vi "Nonredundant Swap Neighborhood.vi"(6 "Number of Machines":i32, 8 "w":i32, 9 "y":i32, 10 "Generate Random indices?":bool, 11 "Schedule in":u16[](array[numeric])) -> (3 "Schedule out":u16[](array[numeric]))   [LabVIEW 2013]
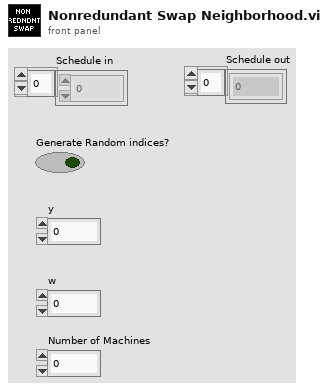
[diagram p1: front panel]
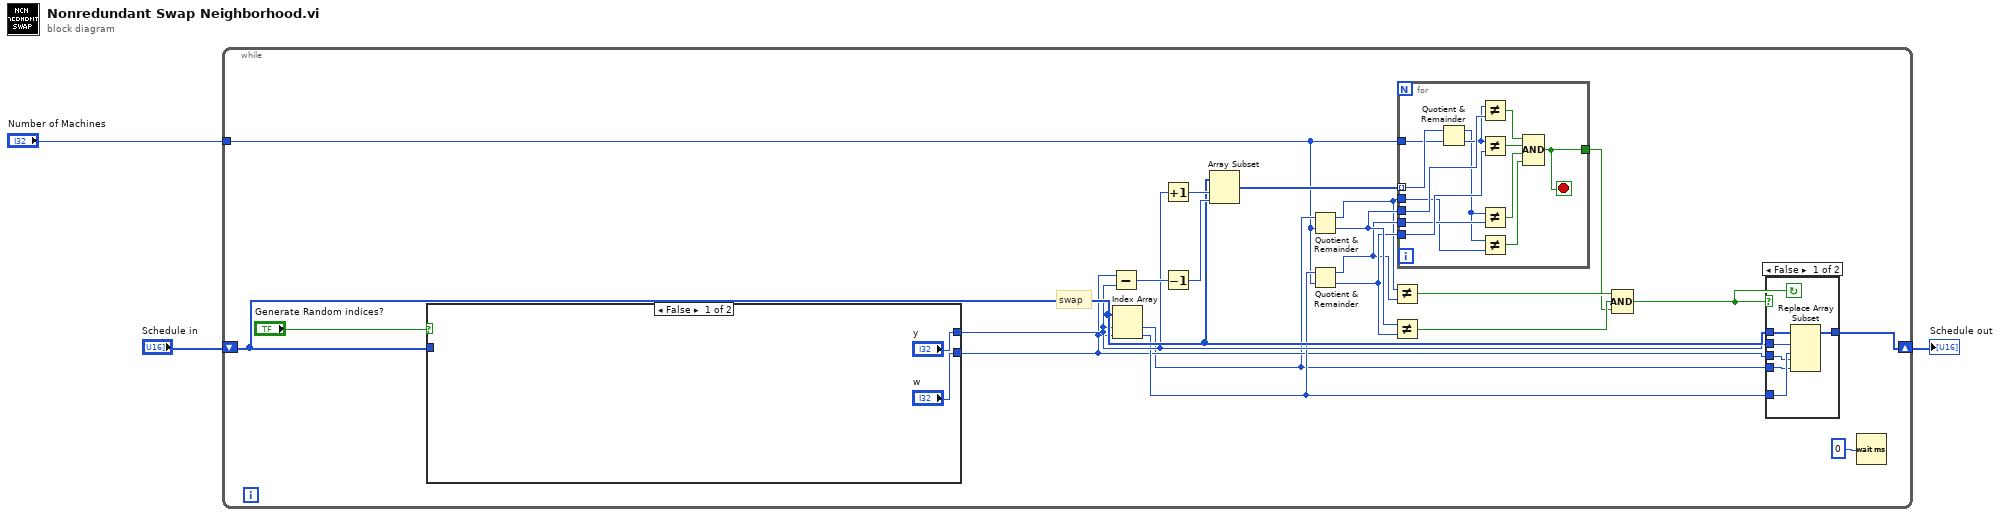
[diagram p0: block diagram]
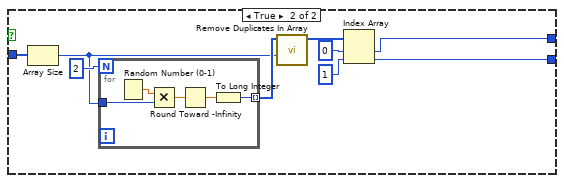
[diagram p2: hidden frame]
diagram:
  n1 = while {
    shift-right: [w11] -> w3
    shift-left: "Schedule in" -> [w12]
    tunnel: "Number of Machines" -> [w6]
    stop <- w13 continue-if-true
    # "swap"
    n2 = case shown="False" "Generate Random indices?" {
      tunnel: w12 -> [_ w32]
      tunnel: ["y" w31] -> w10
      tunnel: ["w" w30] -> w8
      frame False {
      }
      frame True {
        n3 = Array Size(array=w32) -> (size(s)=w28:i32)
        n4 = for {
          N: 2 -> [_]
          tunnel: w28 -> [w37]
          tunnel: [w36] -> w29 mode=indexing
          n5 = Random Number (0-1)() -> (number: 0 to 1=w40:dbl)
          n6 = Multiply(x=w40, y=w37) -> (x*y=w39:dbl)
          n7 = Round Toward -Infinity(1:w39) -> (0:w38:dbl)
          n8 = To Long Integer(number=w38) -> (32bit integer=w36:i32)
        }
        n9 = call "Remove Duplicates In Array.vi"("Max Index Bound"=w28, "Random Numbers Array"=w29) -> ("Random Numbers Array without Duplicates"=w27:i32[])  [unwired: 9 in]
        n10 = Index Array(array=w27, index #1=0 ("index"), index #2=1 ("index")) -> (element #1=w31:i32, element #2=w30:i32)
      }
    }
    n11 = Subtract(x=w8, y=w10) -> (x-y=w21:i32)
    n12 = Index Array(array=w12, index #1=w10, index #2=w8) -> (element #1=w7:u16, element #2=w9:u16)
    n13 = Increment(x=w10) -> (x+1=w22:i32)
    n14 = Decrement(x=w21) -> (x-1=w20:i32)
    n15 = Array Subset(array=w12, index=w22, length=w20) -> (w19:u16[])
    n16 = Quotient & Remainder(x=w7, y=w6) -> (x-y*floor(x/y)=w15:i32, floor(x/y)=w18:i32)
    n17 = Quotient & Remainder(x=w9, y=w6) -> (x-y*floor(x/y)=w16:i32, floor(x/y)=w17:i32)
    n18 = Not Equal?(x=w15, y=w16) -> (x != y?=w24:bool)
    n19 = Not Equal?(x=w18, y=w17) -> (x != y?=w23:bool)
    n20 = for {
      tunnel: w19 -> [w60] mode=indexing
      tunnel: w6 -> [w59]
      tunnel: w18 -> [w58]
      tunnel: w17 -> [w57]
      tunnel: w16 -> [w55]
      tunnel: w15 -> [w54]
      tunnel: [w48] -> w14
      stop <- w48 stop-if-true
      n21 = Quotient & Remainder(x=w60, y=w59) -> (x-y*floor(x/y)=w53:i32, floor(x/y)=w56:i32)
      n22 = Not Equal?(x=w56, y=w58) -> (x != y?=w52:bool)
      n23 = Not Equal?(x=w56, y=w57) -> (x != y?=w51:bool)
      n24 = Not Equal?(x=w53, y=w55) -> (x != y?=w50:bool)
      n25 = Not Equal?(x=w53, y=w54) -> (x != y?=w49:bool)
      n26 = Compound Arithmetic op=AND(w52, w51, w50, w49) -> (w48:bool)
    }
    n27 = Compound Arithmetic op=AND(w24, w23, w14) -> (w13:bool)
    n28 = case shown="False" w13 {
      tunnel: w12 -> [w46 w47]
      tunnel: [w41 w47] -> w11
      tunnel: w10 -> [w45 _]
      tunnel: w9 -> [w44 _]
      tunnel: w8 -> [w43 _]
      tunnel: w7 -> [w42 _]
      frame False {
        n29 = Replace Array Subset(array=w46, new element #1=w44, index #1=w45, new element #2=w42, index #2=w43) -> (w41:u16[])
      }
      frame True {
      }
    }
    n30 = Wait (ms)(milliseconds to wait=u32 0) -> ()  [unwired: 1 out]
  }
  "Schedule out" <- w3
